vi "Drive PID.vi"(11 "Process Variable":dbl format="%.2f") -> (3 "Output":dbl format="%.2f")   [LabVIEW 2013]
uses:
  <vilib>/Rock Robotics/WPI/DriverStation/WPI_DriverStationRobotMode2.ctl
  Begin/Robot Global Data.vi
  <vilib>/addons/control/pid/pid.llb/PID (DBL).vi
  <vilib>/addons/control/pid/NI_PID_pid.lvlib
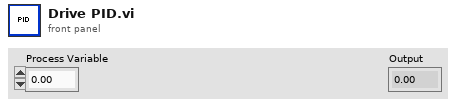
[diagram p1: front panel]
types:
  T1 = typedef "WPI_DriverStationRobotMode2.ctl" = enum16{"Autonomous Disabled", "Autonomous Enabled", "Teleop Disabled", "Teleop Enabled", "Timeout", "Finish", "Test Disabled", "Test Enabled"}
  T2 = cluster{"proportional gain (Kc)":dbl, "integral time (Ti, min)":dbl, "derivative time (Td, min)":dbl}
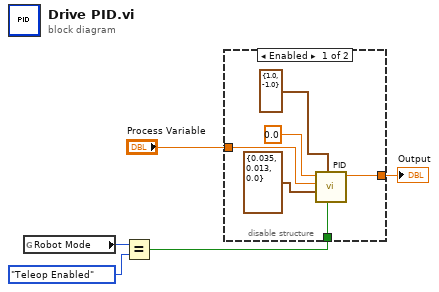
[diagram p0: block diagram]
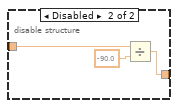
[diagram p2: hidden frame]
diagram:
  n1 = global read "Robot Global Data.vi" "Robot Mode"() -> (w2:T1)
  n2 = Equal?(x=w2, y=WPI_DriverStationRobotMode2."Teleop Enabled" ("Robot Mode")) -> (x = y?=w1:bool)
  n3 = disable-structure shown="Enabled" {
    disable-tunnel: "Process Variable" -> [w9 w14]
    disable-tunnel: [w7 w12] -> w4
    disable-tunnel: w1 -> [w6 _]
    frame Enabled {
      n4 = call-poly <vilib>:"PID.vi"("reinitialize? (F)"=w6, "output range"=cluster{"output high":dbl, "output low":dbl} {"output high"=1.0, "output low"=-1.0}, "PID gains"=T2 {"proportional gain (Kc)"=0.035, "integral time (Ti, min)"=0.013, "derivative time (Td, min)"=0.0}, "process variable"=w9, "setpoint"=0.0) -> ("output"=w7:dbl)  [unwired: 5 in, 1 out]
    }
    frame Disabled {
      n5 = Divide(x=w14, y=-90.0) -> (x/y=w12:dbl)
    }
  }
  "Output" <- w4
